vi "Read Settings.vi"(8 "error in (no error)":errorcluster, 11 "LakeShore370 in":refnum<class "LakeShore370_device.lvclass">) -> (0 "error out":errorcluster, 2 "Settings":string, 3 "LakeShore370 out":refnum<class "LakeShore370_device.lvclass">)   [LabVIEW 2015, in "LakeShore370_device.lvclass"]
uses:
  LakeShore370_device.lvclass
  Instrument/Instrument.lvclass
  Instrument with scanner/Instrument with scanner.lvclass
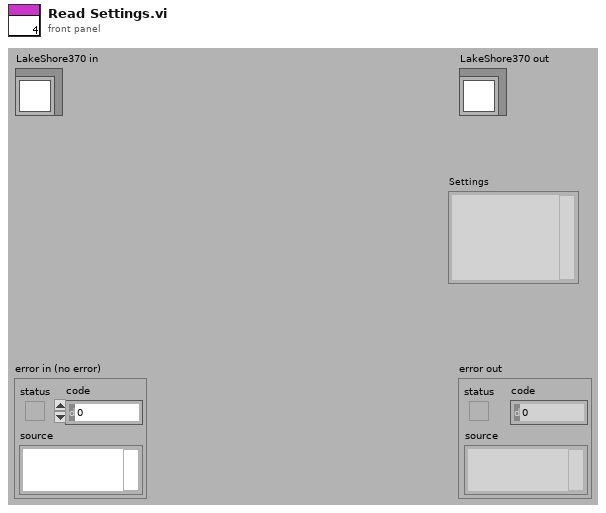
[diagram p1: front panel]
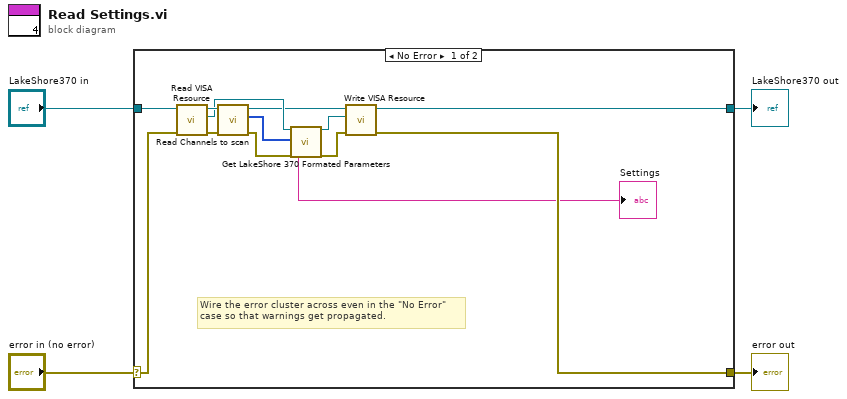
[diagram p0: block diagram]
diagram:
  n1 = case shown="No Error" "error in (no error)" {
    selector: "error in (no error)" -> [w14 w19]
    tunnel: [w12 w19] -> w3
    tunnel: [w15 w18] -> w1
    tunnel: "LakeShore370 in" -> [w17 w18]
    frame No Error {
      # "Wire the error cluster across even in the \"No Error\"\ncase so that warnings get propagated."
      n2 = call "Read VISA Resource.vi"("error in (no error)"=w14, "Instrument.lvclass in"=w17) -> ("error out"=w8:errorcluster, "VISA Resource"=w11:refnum<visa-resource-name>, "Instrument.lvclass out"=w16:refnum<class "LakeShore370_device.lvclass">)  [unwired: 7 out]
      n3 = call "Read Channels to scan.vi"("error in (no error)"=w8, "Instrument with scanner.lvclass in"=w16) -> ("error out"=w7:errorcluster, "Channels to scan (empty - don't use scanner option)"=w6:i32[], "Instrument with scanner.lvclass out"=w9:refnum<class "LakeShore370_device.lvclass">)  [unwired: 7 out]
      n4 = call "Get LakeShore 370 Formated Parameters.vi"("VISA Resource Name"=w11, "Channels to scan (empty - don't use scanner option)"=w6, "error in (no error)"=w7) -> ("Parameters"=→"Settings":string, "VISA Resource Name Out"=w10:refnum<visa-resource-name>, "error out"=w13:errorcluster)  [unwired: 1 in, 13 out]
      n5 = call "Write VISA Resource.vi"("error in (no error)"=w13, "VISA Resource"=w10, "Instrument.lvclass in"=w9) -> ("error out"=w12:errorcluster, "Instrument.lvclass out"=w15:refnum<class "LakeShore370_device.lvclass">)  [unwired: 7 out]
    }
    frame Error {
    }
  }
  "error out" <- w3
  "LakeShore370 out" <- w1
